vi "Resideo String Data.vi"(11 "Vesta LDO":T1) -> (3 "Vesta Data":string[][](array[string]))   [LabVIEW 2020]
uses:
  Type Definitions/Vesta Info.ctl
panel:
  out "error out":errorcluster
  in  "error in (no error)":errorcluster
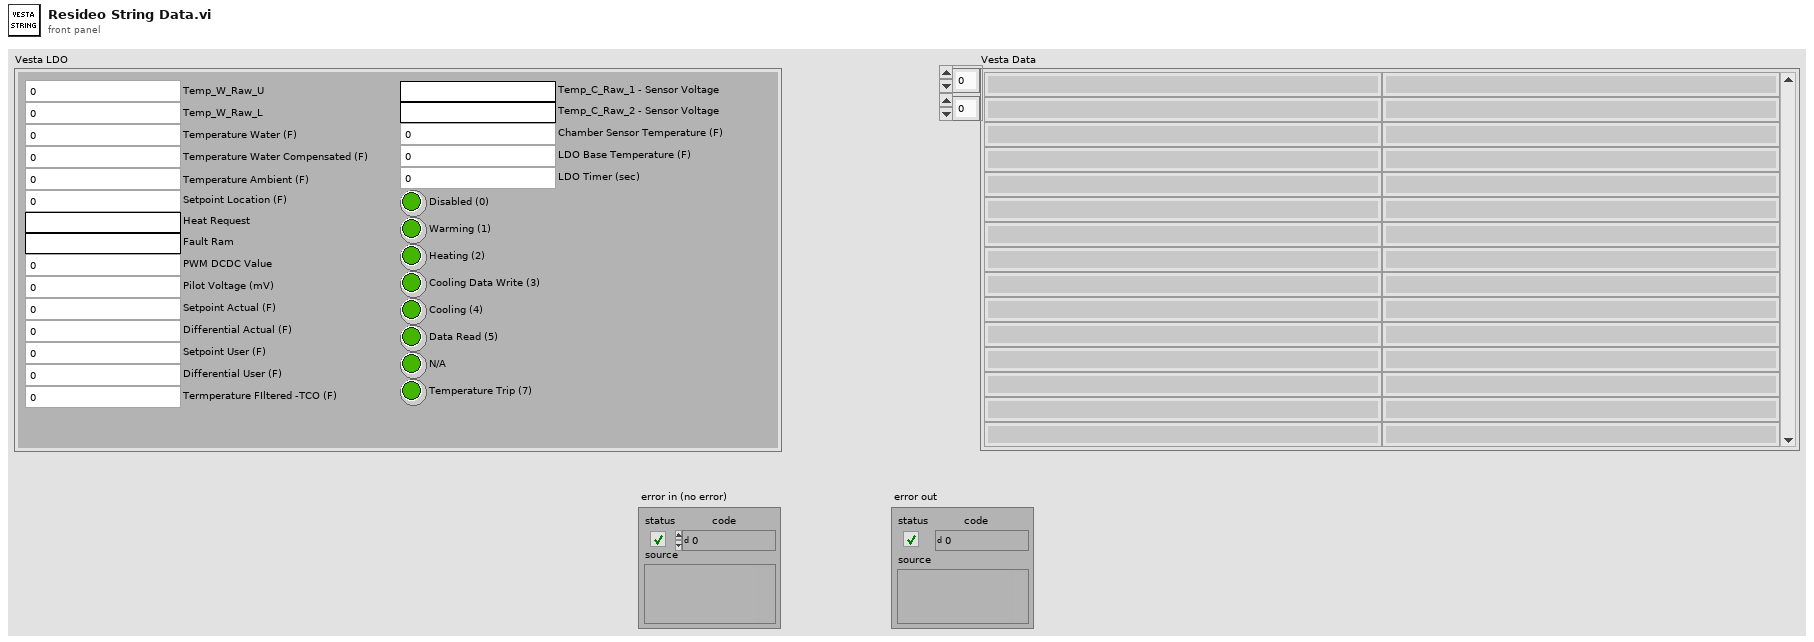
[diagram p1: front panel]
types:
  T1 = typedef "Vesta Info.ctl" = cluster{"Temp_W_Raw_U":u16, "Temp_W_Raw_L":u16, "Temperature Water (F)":dbl, "Temperature Water Compensated (F)":dbl, "Temperature Ambient (F)":dbl, "Setpoint Location (F)":dbl, "Heat Request":string, "Fault Ram":string, "PWM DCDC Value":u16, "Pilot Voltage (mV)":dbl, "Setpoint Actual (F)":dbl, "Differential Actual (F)":dbl, "Setpoint User (F)":dbl, "Differential User (F)":dbl, "Termperature FIltered -TCO (F)":dbl, "Temp_C_Raw_1 - Sensor Voltage":string, "Temp_C_Raw_2 - Sensor Voltage":string, "Chamber Sensor Temperature (F)":dbl, "LDO Base Temperature (F)":dbl, "LDO Timer (sec)":i16, "Disabled (0)":bool, "Warming (1)":bool, "Heating (2)":bool, "Cooling Data Write (3)":bool, "Cooling (4)":bool, "Data Read (5)":bool, "N/A":bool, "Temperature Trip (7)":bool}
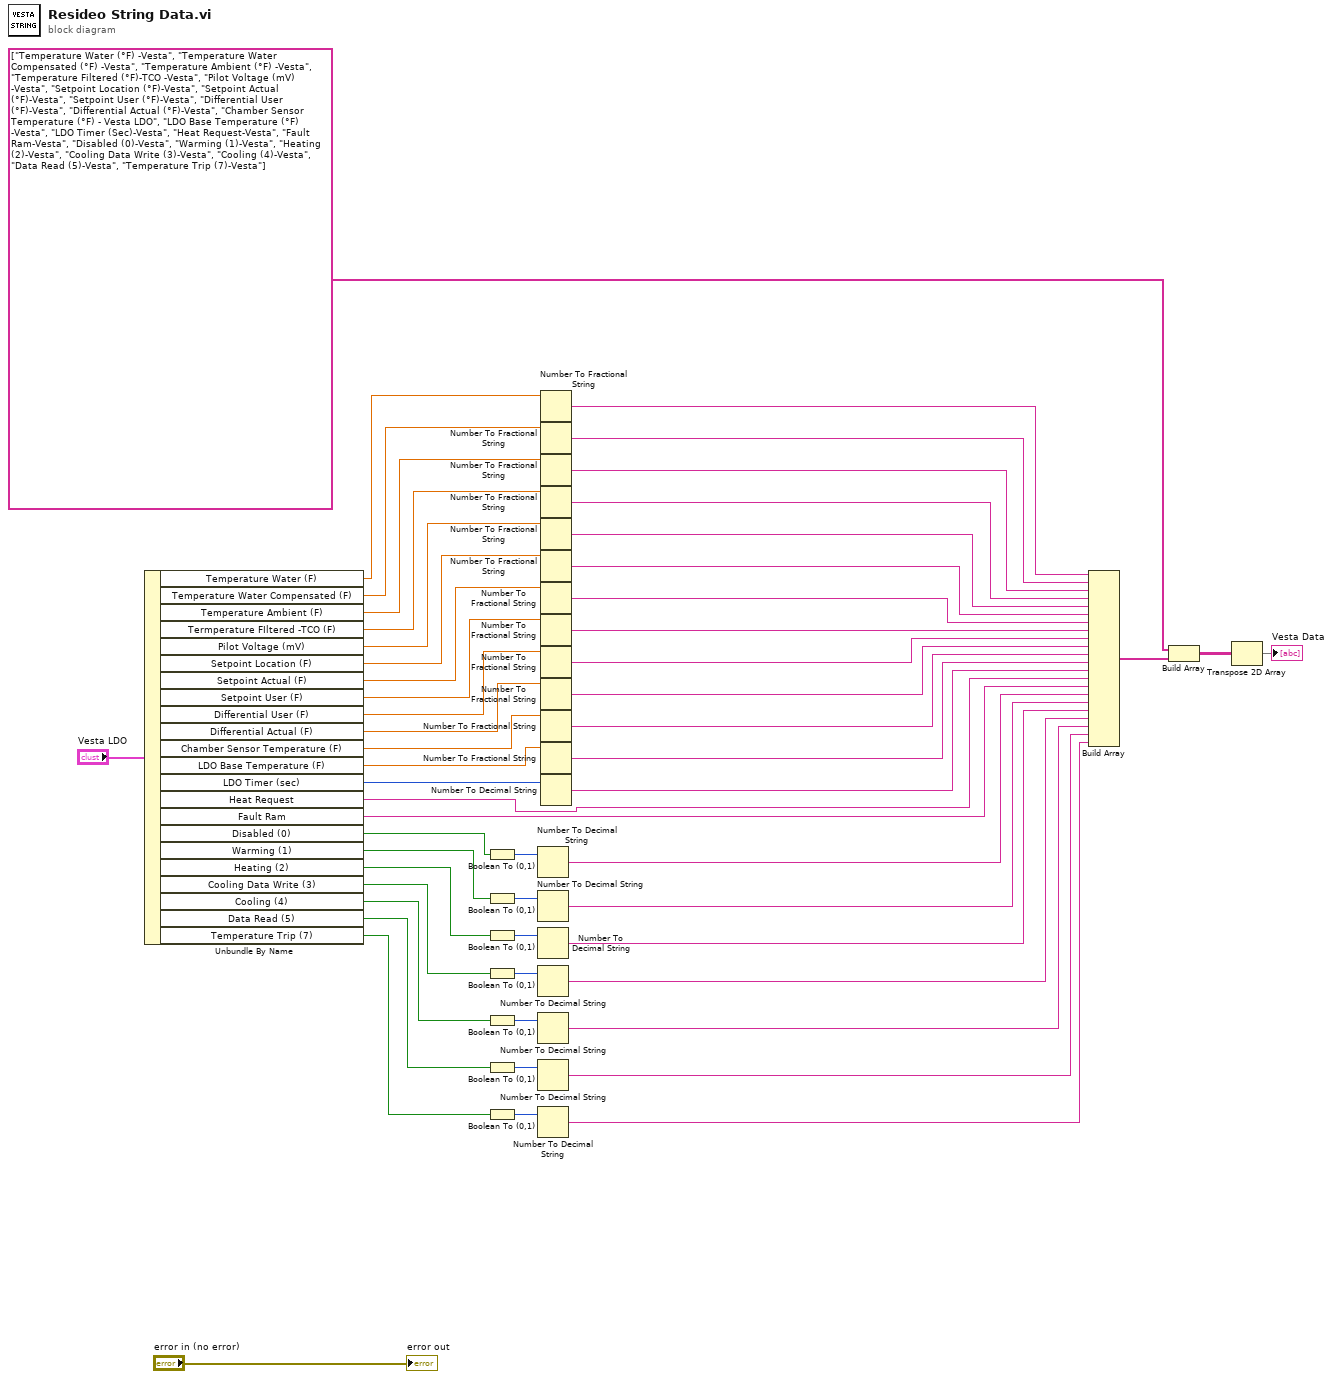
[diagram p0: block diagram]
diagram:
  n1 = Unbundle By Name("Vesta LDO") -> ("Temperature Water (F)"=w53:dbl, "Temperature Water Compensated (F)"=w52:dbl, "Temperature Ambient (F)"=w51:dbl, "Termperature FIltered -TCO (F)"=w50:dbl, "Pilot Voltage (mV)"=w49:dbl, "Setpoint Location (F)"=w48:dbl, "Setpoint Actual (F)"=w47:dbl, "Setpoint User (F)"=w46:dbl, "Differential User (F)"=w45:dbl, "Differential Actual (F)"=w44:dbl, "Chamber Sensor Temperature (F)"=w43:dbl, "LDO Base Temperature (F)"=w42:dbl, "LDO Timer (sec)"=w41:i16, "Heat Request"=w13:string, "Fault Ram"=w12:string, "Disabled (0)"=w40:bool, "Warming (1)"=w39:bool, "Heating (2)"=w38:bool, "Cooling Data Write (3)"=w37:bool, "Cooling (4)"=w36:bool, "Data Read (5)"=w35:bool, "Temperature Trip (7)"=w34:bool)
  n2 = Boolean To (0,1)(Boolean=w40) -> (0, 1=w33:i16)
  n3 = Boolean To (0,1)(Boolean=w39) -> (0, 1=w32:i16)
  n4 = Boolean To (0,1)(Boolean=w38) -> (0, 1=w31:i16)
  n5 = Boolean To (0,1)(Boolean=w37) -> (0, 1=w30:i16)
  n6 = Boolean To (0,1)(Boolean=w36) -> (0, 1=w29:i16)
  n7 = Boolean To (0,1)(Boolean=w35) -> (0, 1=w28:i16)
  n8 = Boolean To (0,1)(Boolean=w34) -> (0, 1=w27:i16)
  n9 = Number To Decimal String(number=w33) -> (decimal integer string=w11:string)  [unwired: 1 in]
  n10 = Number To Decimal String(number=w32) -> (decimal integer string=w10:string)  [unwired: 1 in]
  n11 = Number To Decimal String(number=w31) -> (decimal integer string=w9:string)  [unwired: 1 in]
  n12 = Number To Decimal String(number=w30) -> (decimal integer string=w8:string)  [unwired: 1 in]
  n13 = Number To Decimal String(number=w29) -> (decimal integer string=w7:string)  [unwired: 1 in]
  n14 = Number To Decimal String(number=w28) -> (decimal integer string=w6:string)  [unwired: 1 in]
  n15 = Number To Decimal String(number=w27) -> (decimal integer string=w5:string)  [unwired: 1 in]
  n16 = Number To Fractional String(number=w53) -> (F-format string=w26:string)  [unwired: 3 in]
  n17 = Number To Fractional String(number=w52) -> (F-format string=w25:string)  [unwired: 3 in]
  n18 = Number To Fractional String(number=w51) -> (F-format string=w24:string)  [unwired: 3 in]
  n19 = Number To Fractional String(number=w50) -> (F-format string=w23:string)  [unwired: 3 in]
  n20 = Number To Fractional String(number=w49) -> (F-format string=w22:string)  [unwired: 3 in]
  n21 = Number To Fractional String(number=w48) -> (F-format string=w21:string)  [unwired: 3 in]
  n22 = Number To Fractional String(number=w47) -> (F-format string=w20:string)  [unwired: 3 in]
  n23 = Number To Fractional String(number=w46) -> (F-format string=w19:string)  [unwired: 3 in]
  n24 = Number To Fractional String(number=w45) -> (F-format string=w18:string)  [unwired: 3 in]
  n25 = Number To Fractional String(number=w44) -> (F-format string=w17:string)  [unwired: 3 in]
  n26 = Number To Fractional String(number=w43) -> (F-format string=w16:string)  [unwired: 3 in]
  n27 = Number To Fractional String(number=w42) -> (F-format string=w15:string)  [unwired: 3 in]
  n28 = Number To Decimal String(number=w41) -> (decimal integer string=w14:string)  [unwired: 1 in]
  n29 = Build Array(w26, w25, w24, w23, w22, w21, w20, w19, w18, w17, w16, w15, w14, w13, w12, w11, w10, w9, w8, w7, w6, w5) -> (w4:string[])
  n30 = Build Array(string[] ["Temperature Water (°F) -Vesta", "Temperature Water Compensated (°F) -Vesta", "Temperature Ambient (°F) -Vesta", "Temperature Filtered (°F)-TCO -Vesta", "Pilot Voltage (mV) -Vesta", "Setpoint Location (°F)-Vesta", "Setpoint Actual (°F)-Vesta", "Setpoint User (°F)-Vesta", "Differential User (°F)-Vesta", "Differential Actual (°F)-Vesta", "Chamber Sensor Temperature (°F) - Vesta LDO", "LDO Base Temperature (°F) -Vesta", "LDO Timer (Sec)-Vesta", "Heat Request-Vesta", "Fault Ram-Vesta", "Disabled (0)-Vesta", "Warming (1)-Vesta", "Heating (2)-Vesta", "Cooling Data Write (3)-Vesta", "Cooling (4)-Vesta", "Data Read (5)-Vesta", "Temperature Trip (7)-Vesta"], w4) -> (w2:string[][])
  n31 = Transpose 2D Array(2D array=w2) -> (transposed array=→"Vesta Data":string[][])
  "error out" <- "error in (no error)"
